vi "GPS NMEA Checksum_sub.vi"(1 "Raw Sentence":string) -> (0 "유효?":bool)   [LabVIEW 2015]
panel:
  out "ref CheckSum":u8 format="%x"
  out "CheckSum":u8 format="%x"
  out "Sentence":string
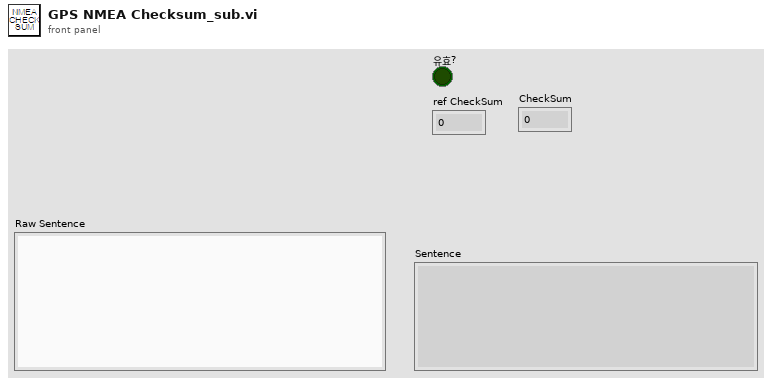
[diagram p1: front panel]
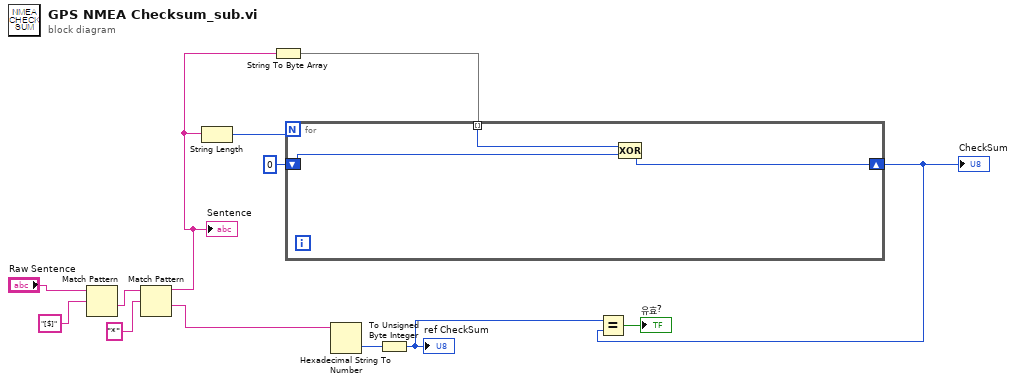
[diagram p0: block diagram]
diagram:
  n1 = Match Pattern(string="Raw Sentence", regular expression="[$]" ("검색 문자열/문자 (-)")) -> (after substring=w10:string)  [unwired: 1 in, 3 out]
  n2 = Match Pattern(string=w10, regular expression="*" ("정규식")) -> (before substring=w8:string, after substring=w3:string)  [unwired: 1 in, 2 out]
  "Sentence" <- w8
  n3 = String Length(string=w8) -> (length=w9:i32)
  n4 = String To Byte Array(string=w8) -> (unsigned byte array=w7:u8[])
  n5 = for {
    N: w9 -> [_]
    shift-right: [w16] -> w5
    shift-left: u8 0 -> [w15]
    tunnel: w7 -> [w14] mode=indexing
    n6 = Compound Arithmetic op=XOR ("복합 연산")(w14, w15) -> (w16:u8)
  }
  "CheckSum" <- w5
  n7 = Hexadecimal String To Number(string=w3) -> (number=w2:u32)  [unwired: 2 in, 1 out]
  n8 = To Unsigned Byte Integer(number=w2) -> (unsigned 8bit integer=w1:u8)
  "ref CheckSum" <- w1
  n9 = Equal?(x=w1, y=w5) -> (x = y?=→"유효?":bool)
